vi "lab session 7.1.vi"() -> ()   [LabVIEW 2020]
panel:
  out "x*y":dbl[](array[numeric])
  out "subarray":dbl[](array[numeric])
  in  "# of elements":i32
  in  "start subset":i32
  in  "y":dbl
  out "x":dbl[](array[numeric])
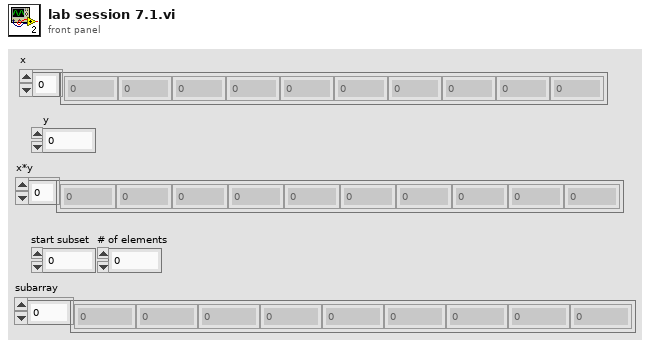
[diagram p1: front panel]
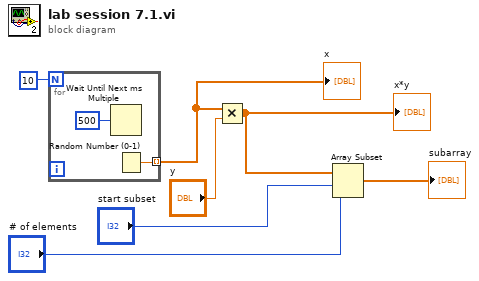
[diagram p0: block diagram]
diagram:
  n1 = for {
    N: 10 -> [_]
    tunnel: [w8] -> w2 mode=indexing
    n2 = Wait Until Next ms Multiple(millisecond multiple=u32 500) -> ()  [unwired: 1 out]
    n3 = Random Number (0-1)() -> (number: 0 to 1=w8:dbl)
  }
  "x" <- w2
  n4 = Multiply(x=w2, y="y") -> (x*y=w1:dbl[])
  "x*y" <- w1
  n5 = Array Subset(array=w1, index="start subset", length="# of elements") -> (→"subarray":dbl[])
